vi "Enter Sample Weight (SubVI).vi"(0 "Weight Ref":refnum<vi>, 7 "References":T1) -> ()   [LabVIEW 2010]
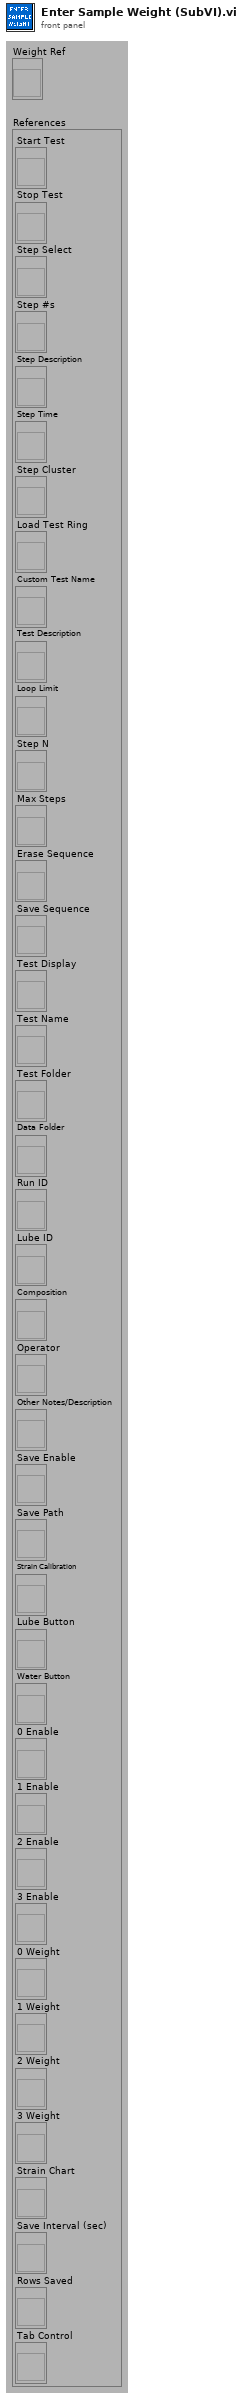
[diagram p1: front panel]
types:
  T1 = cluster{"Start Test":refnum<vi>, "Stop Test":refnum<vi>, "Step Select":refnum<vi>, "Step #s":refnum<vi>, "Step Description":refnum<vi>, "Step Time":refnum<vi>, "Step Cluster":refnum<vi>, "Load Test Ring":refnum<vi>, "Custom Test Name":refnum<vi>, "Test Description":refnum<vi>, "Loop Limit":refnum<vi>, "Step N":refnum<vi>, "Max Steps":refnum<vi>, "Erase Sequence":refnum<vi>, "Save Sequence":refnum<vi>, "Test Display":refnum<vi>, "Test Name":refnum<vi>, "Test Folder":refnum<vi>, "Data Folder":refnum<vi>, "Run ID":refnum<vi>, "Lube ID":refnum<vi>, "Composition":refnum<vi>, "Operator":refnum<vi>, "Other Notes/Description":refnum<vi>, "Save Enable":refnum<vi>, "Save Path":refnum<vi>, "Strain Calibration":refnum<vi>, "Lube Button":refnum<vi>, "Water Button":refnum<vi>, "0 Enable":refnum<vi>, "1 Enable":refnum<vi>, "2 Enable":refnum<vi>, "3 Enable":refnum<vi>, "0 Weight":refnum<vi>, "1 Weight":refnum<vi>, "2 Weight":refnum<vi>, "3 Weight":refnum<vi>, "Strain Chart":refnum<vi>, "Save Interval (sec)":refnum<vi>, "Rows Saved":refnum<vi>, "Tab Control":refnum<vi>}
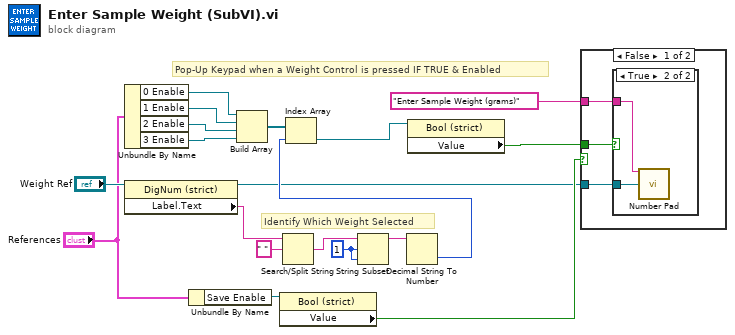
[diagram p0: block diagram]
diagram:
  w5 = 1
  # "Pop-Up Keypad when a Weight Control is pressed IF TRUE & Enabled"
  # "Identify Which Weight Selected"
  n1 = Unbundle By Name("References") -> ("0 Enable"=w9:refnum<vi>, "1 Enable"=w3:refnum<vi>, "2 Enable"=w2:refnum<vi>, "3 Enable"=w1:refnum<vi>)
  n2 = property class="DigNum (strict)"(reference="Weight Ref") -> (reference out=w13:refnum<vi>, "Label.Text"=w8:string)  [unwired: 1 in, 1 out]
  n3 = Unbundle By Name("References") -> ("Save Enable"=w16:refnum<vi>)
  n4 = Build Array(w9, w3, w2, w1) -> (w10:refnum<vi>[])
  n5 = property class="Bool (strict)"(reference=w16) -> ("Value"=w17:bool)  [unwired: 1 in, 2 out]
  n6 = Search/Split String(string=w8, search string/char (-)=" ") -> (match + rest of string=w6:string)  [unwired: 1 in, 2 out]
  n7 = String Subset(string=w6, offset (0)=w5, length (rest)=w5) -> (substring=w7:string)
  n8 = Decimal String To Number(string=w7) -> (number=w15:i32)  [unwired: 2 in, 1 out]
  n9 = Index Array(array=w10, index=w15) -> (element=w11:refnum<vi>)
  n10 = property class="Bool (strict)"(reference=w11) -> ("Value"=w12:bool)  [unwired: 1 in, 2 out]
  n11 = case shown="False" w17 {
    tunnel: w12 -> [w22 _]
    tunnel: w13 -> [w21 _]
    tunnel: "Enter Sample Weight (grams)" ("Instruction") -> [w20 _]
    frame False {
      n12 = case shown="True" w22 {
        tunnel: w21 -> [_ w24]
        tunnel: w20 -> [_ w23]
        frame False {
        }
        frame True {
          n13 = call "Number Pad.vi"("Instruction"=w23, "CtlRef"=w24) -> ()  [unwired: 11 in, 3 out]
        }
      }
    }
    frame True {
    }
  }
